vi "Remove JSON Tag.vi"(11 "Name":string) -> (2 "tagged as JSON text":bool, 3 "Name (tag stripped)":string)   [LabVIEW 2015, in "JSONtext.lvlib"]
uses:
  JSONtext.lvlib
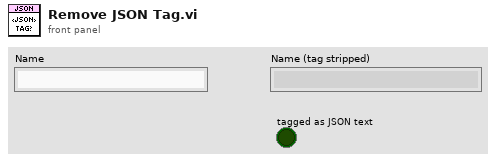
[diagram p1: front panel]
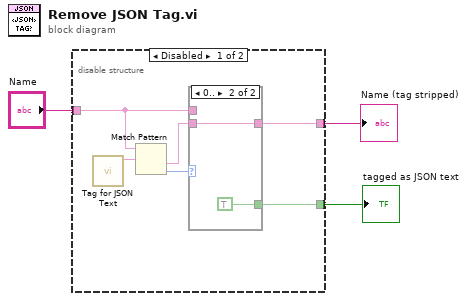
[diagram p0: block diagram]
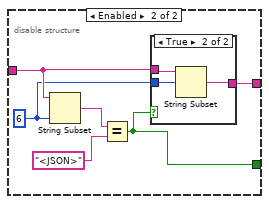
[diagram p3: hidden frame]
diagram:
  n1 = disable-structure shown="Disabled" {
    disable-tunnel: [w9 w16] -> w3
    disable-tunnel: "Name" -> [w5 w14]
    disable-tunnel: [w4 w15] -> w1
    frame Disabled {
      n2 = call "Tag for JSON Text.vi"() -> ("Tag for JSON text"=w6:string)  [unwired: 11 in]
      n3 = Match Pattern(string=w5, regular expression=w6) -> (after substring=w7:string, offset past match=w8:i32)  [unwired: 1 in, 2 out]
      n4 = case shown="0.." w8 {
        tunnel: [w10 w11] -> w4
        tunnel: w5 -> [w10 _]
        tunnel: w7 -> [_ w11]
        tunnel: [_ TRUE] -> w9
        frame ..-1 {
        }
        frame 0.. {
        }
      }
    }
    frame Enabled {
      w13 = 6 ("length (rest)")
      n5 = String Subset(string=w14, length (rest)=w13) -> (substring=w18:string)  [unwired: 1 in]
      n6 = Equal?(x=w18, y="<JSON>") -> (x = y?=w16:bool)
      n7 = case shown="True" w16 {
        tunnel: [w19 w21] -> w15
        tunnel: w14 -> [w19 w22]
        tunnel: w13 -> [_ w20]
        frame False {
        }
        frame True {
          n8 = String Subset(string=w22, offset (0)=w20) -> (substring=w21:string)  [unwired: 1 in]
        }
      }
    }
  }
  "tagged as JSON text" <- w3
  "Name (tag stripped)" <- w1
